vi "Validate Configuration.vi"(8 "error in (no error)":errorcluster, 11 "Numeric Limit Compare Config in":refnum<class "Numeric Limit Compare Config.lvclass">) -> (0 "error out":errorcluster, 3 "Numeric Limit Compare Config out":refnum<class "Numeric Limit Compare Config.lvclass">)   [LabVIEW 2015, in "Numeric Limit Compare Config.lvclass"]
doc: "This function performs validation of the configuration. This function should be safe to call at any point and should not rely on anything in the runtime environment."
uses:
  Numeric Limit Compare Config.lvclass
  <vilib>/NI/Tag Bus/tag/Data Type.ctl
  <vilib>/NI/Tag Bus Module Framework/channel/channel classification.ctl
  Numeric Limit Compare Config.lvclass/Numeric Limit Compare Config.ctl
  <vilib>/NI/Tag Bus/tag/tag descriptor.lvclass/tag descriptor.ctl
  <vilib>/NI/Tag Bus Module Framework/channel/TBM channel.lvclass/TBM channel.ctl
  <vilib>/NI/Tag Bus/tag/tag descriptor.lvclass
  <vilib>/NI/Tag Bus Module Framework/channel/TBM channel.lvclass
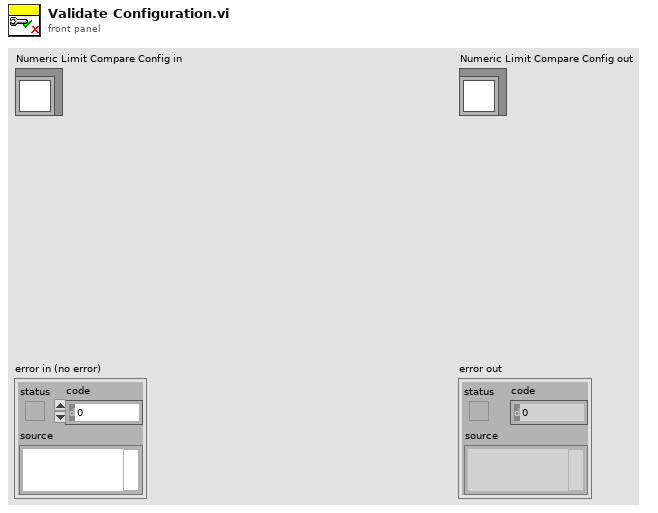
[diagram p1: front panel]
types:
  T1 = typedef "TBM channel.lvclass/channel classification.ctl" = enum16{"input data", "output data", "processing parameter", "processing result"}
  T2 = typedef "tag bus.lvlib/tag descriptor.lvclass/Data Type.ctl" = enum16{"Double", "Single", "I64", "I32", "I16", "I8", "U64", "U32", "U16", "U8", "Boolean", "String", "Array of Double", "Array of Single", "Array of I64", "Array of I32", "Array of I16", "Array of I8", "Array of U64", "Array of U32", "Array of U16", "Array of U8", "Array of Boolean", "Array of String"}
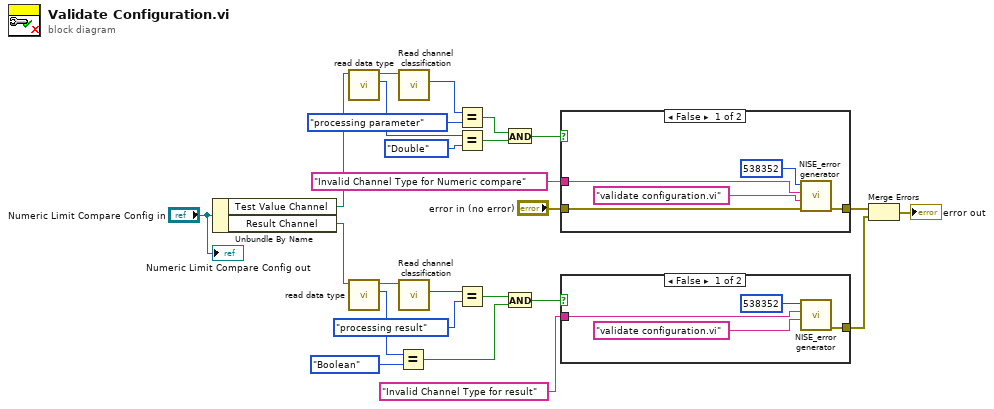
[diagram p0: block diagram]
diagram:
  n1 = Unbundle By Name("Numeric Limit Compare Config in") -> ("Test Value Channel"=w25:refnum<class "TBM channel.lvclass">, "Result Channel"=w20:refnum<class "TBM channel.lvclass">)
  n2 = call <vilib>:"read data type.vi"("system tag in"=w25) -> ("data type"=w24:T2, "system tag out"=w13:refnum<class "TBM channel.lvclass">)  [unwired: 8 in, 1 out]
  n3 = call <vilib>:"read data type.vi"("system tag in"=w20) -> ("data type"=w14:T2, "system tag out"=w9:refnum<class "TBM channel.lvclass">)  [unwired: 8 in, 1 out]
  n4 = Equal?(x=w14, y=Data_Type."Boolean") -> (x = y?=w18:bool)
  n5 = call <vilib>:"Read channel classification.vi"("channel in"=w13) -> ("channel classification"=w12:T1)  [unwired: 8 in, 2 out]
  n6 = call <vilib>:"Read channel classification.vi"("channel in"=w9) -> ("channel classification"=w10:T1)  [unwired: 8 in, 2 out]
  n7 = Equal?(x=w12, y=channel_classification."processing parameter") -> (x = y?=w5:bool)
  n8 = Equal?(x=w24, y=Data_Type."Double") -> (x = y?=w22:bool)
  n9 = Equal?(x=w10, y=channel_classification."processing result") -> (x = y?=w4:bool)
  n10 = And(x=w5, y=w22) -> (x .and. y?=w6:bool)
  n11 = And(x=w4, y=w18) -> (x .and. y?=w7:bool)
  n12 = case shown="False" w6 {
    tunnel: [w30 w31] -> w16
    tunnel: "Invalid Channel Type for Numeric compare" ("accessors:name") -> [w29 _]
    tunnel: "error in (no error)" -> [w26 w31]
    frame False {
      n13 = call <vilib>:"NISE_error generator.vi"("error in"=w26, "source"="validate configuration.vi" ("format string"), "append error message"=w29, "error code (0)"=538352) -> ("error out"=w30:errorcluster)  [unwired: 5 in]
    }
    frame True {
    }
  }
  n14 = case shown="False" w7 {
    tunnel: [w35 _] -> w15
    tunnel: "Invalid Channel Type for result" ("accessors:name") -> [w34 _]
    frame False {
      n15 = call <vilib>:"NISE_error generator.vi"("source"="validate configuration.vi" ("format string"), "append error message"=w34, "error code (0)"=538352) -> ("error out"=w35:errorcluster)  [unwired: 6 in]
    }
    frame True {
    }
  }
  n16 = Merge Errors(w16, w15) -> (→"error out":errorcluster)
  "Numeric Limit Compare Config out" <- "Numeric Limit Compare Config in"
